vi "niWLAN - 80211abgnGeneration(ref).vi"(0 "Waveform Generation Settings":T1[](array[typedef])=[{"Standard"=0, "Channel Bandwidth (Hz)"=20000000.0, "Idle Interval (s)"=0.0001, "MCS Index"=0, "80211n PLCP Frame Format"=0, "Payload Data Length (bytes)"=100, "OFDM Data Rate (Mbps)"=0, "DSSS Data Rate (Mbps)"=0, "Wfm_Index"=0}, {"Standard"=0, "Channel Bandwidth (Hz)"=20000000.0, "Idle Interval (s)"=0.001, "MCS Index"=0, "80211n PLCP Frame Format"=0, "Payload Data Length (bytes)"=200, "OFDM Data Rate (Mbps)"=2, "DSSS Data Rate (Mbps)"=0, "Wfm_Index"=1}, {"Standard"=0, "Channel Bandwidth (Hz)"=20000000.0, "Idle Interval (s)"=0.0001, "MCS Index"=0, "80211n PLCP Frame Format"=0, "Payload Data Length (bytes)"=300, "OFDM Data Rate (Mbps)"=4, "DSSS Data Rate (Mbps)"=0, "Wfm_Index"=2}, {"Standard"=0, "Channel Bandwidth (Hz)"=20000000.0, "Idle Interval (s)"=0.0001, "MCS Index"=0, "80211n PLCP Frame Format"=0, "Payload Data Length (bytes)"=600, "OFDM Data Rate (Mbps)"=7, "DSSS Data Rate (Mbps)"=0, "Wfm_Index"=3}, {"Standard"=1, "Channel Bandwidth (Hz)"=20000000.0, "Idle Interval (s)"=0.0001, "MCS Index"=0, "80211n PLCP Frame Format"=0, "Payload Data Length (bytes)"=50, "OFDM Data Rate (Mbps)"=0, "DSSS Data Rate (Mbps)"=0, "Wfm_Index"=4}, {"Standard"=1, "Channel Bandwidth (Hz)"=20000000.0, "Idle Interval (s)"=0.0001, "MCS Index"=0, "80211n PLCP Frame Format"=0, "Payload Data Length (bytes)"=200, "OFDM Data Rate (Mbps)"=0, "DSSS Data Rate (Mbps)"=4, "Wfm_Index"=5}, {"Standard"=3, "Channel Bandwidth (Hz)"=20000000.0, "Idle Interval (s)"=0.0001, "MCS Index"=0, "80211n PLCP Frame Format"=0, "Payload Data Length (bytes)"=80, "OFDM Data Rate (Mbps)"=0, "DSSS Data Rate (Mbps)"=0, "Wfm_Index"=6}, {"Standard"=3, "Channel Bandwidth (Hz)"=20000000.0, "Idle Interval (s)"=0.0001, "MCS Index"=4, "80211n PLCP Frame Format"=0, "Payload Data Length (bytes)"=200, "OFDM Data Rate (Mbps)"=0, "DSSS Data Rate (Mbps)"=0, "Wfm_Index"=7}, {"Standard"=3, "Channel Bandwidth (Hz)"=20000000.0, "Idle Interval (s)"=0.0001, "MCS Index"=7, "80211n PLCP Frame Format"=0, "Payload Data Length (bytes)"=700, "OFDM Data Rate (Mbps)"=0, "DSSS Data Rate (Mbps)"=0, "Wfm_Index"=8}, {"Standard"=0, "Channel Bandwidth (Hz)"=20000000.0, "Idle Interval (s)"=0.0001, "MCS Index"=0, "80211n PLCP Frame Format"=0, "Payload Data Length (bytes)"=60, "OFDM Data Rate (Mbps)"=0, "DSSS Data Rate (Mbps)"=0, "Wfm_Index"=9}, {"Standard"=0, "Channel Bandwidth (Hz)"=20000000.0, "Idle Interval (s)"=0.0001, "MCS Index"=0, "80211n PLCP Frame Format"=0, "Payload Data Length (bytes)"=200, "OFDM Data Rate (Mbps)"=2, "DSSS Data Rate (Mbps)"=0, "Wfm_Index"=10}, {"Standard"=0, "Channel Bandwidth (Hz)"=20000000.0, "Idle Interval (s)"=0.0001, "MCS Index"=0, "80211n PLCP Frame Format"=0, "Payload Data Length (bytes)"=300, "OFDM Data Rate (Mbps)"=4, "DSSS Data Rate (Mbps)"=0, "Wfm_Index"=11}, {"Standard"=0, "Channel Bandwidth (Hz)"=20000000.0, "Idle Interval (s)"=0.0001, "MCS Index"=0, "80211n PLCP Frame Format"=0, "Payload Data Length (bytes)"=600, "OFDM Data Rate (Mbps)"=7, "DSSS Data Rate (Mbps)"=0, "Wfm_Index"=12}, {"Standard"=3, "Channel Bandwidth (Hz)"=20000000.0, "Idle Interval (s)"=0.0001, "MCS Index"=0, "80211n PLCP Frame Format"=0, "Payload Data Length (bytes)"=80, "OFDM Data Rate (Mbps)"=0, "DSSS Data Rate (Mbps)"=0, "Wfm_Index"=13}, {"Standard"=3, "Channel Bandwidth (Hz)"=20000000.0, "Idle Interval (s)"=0.0001, "MCS Index"=4, "80211n PLCP Frame Format"=0, "Payload Data Length (bytes)"=300, "OFDM Data Rate (Mbps)"=0, "DSSS Data Rate (Mbps)"=0, "Wfm_Index"=14}, {"Standard"=3, "Channel Bandwidth (Hz)"=20000000.0, "Idle Interval (s)"=0.0001, "MCS Index"=7, "80211n PLCP Frame Format"=0, "Payload Data Length (bytes)"=600, "OFDM Data Rate (Mbps)"=0, "DSSS Data Rate (Mbps)"=0, "Wfm_Index"=15}, {"Standard"=3, "Channel Bandwidth (Hz)"=40000000.0, "Idle Interval (s)"=0.0001, "MCS Index"=0, "80211n PLCP Frame Format"=0, "Payload Data Length (bytes)"=120, "OFDM Data Rate (Mbps)"=0, "DSSS Data Rate (Mbps)"=0, "Wfm_Index"=16}, {"Standard"=3, "Channel Bandwidth (Hz)"=40000000.0, "Idle Interval (s)"=0.0001, "MCS Index"=4, "80211n PLCP Frame Format"=0, "Payload Data Length (bytes)"=400, "OFDM Data Rate (Mbps)"=0, "DSSS Data Rate (Mbps)"=0, "Wfm_Index"=17}, {"Standard"=3, "Channel Bandwidth (Hz)"=40000000.0, "Idle Interval (s)"=0.0001, "MCS Index"=7, "80211n PLCP Frame Format"=0, "Payload Data Length (bytes)"=1024, "OFDM Data Rate (Mbps)"=0, "DSSS Data Rate (Mbps)"=0, "Wfm_Index"=18}] {"DSSS Data Rate (Mbps)" items=["1", "2", "5.5 CCK", "5.5 PBCC", "11 CCK", "11 PBCC", "22", "33"]; "OFDM Data Rate (Mbps)" items=["6", "9", "12", "18", "24", "36", "48", "54"]; "80211n PLCP Frame Format" items=["Mixed Format", "Greenfield Format"]; "Standard" items=["80211A/G/J/P OFDM", "80211B/G DSSS", "80211G DSSSOFDM", "80211N MIMOOFDM", "80211AC MIMOOFDM"]}, 5 "Without ACK ?":bool, 7 "Address String":string="00:90:4C:C5:12:38", 11 "error in":errorcluster) -> (4 "Output":T2(array[cluster]), 15 "error out":errorcluster)   [LabVIEW 2011]
uses:
  TV/RW/Includes/WLAN - TV - RW - INC - Rx_PER_Wfm_Settings.ctl
  <vilib>/RF Toolkits/WLAN/generation/controls/wlanG version control.ctl
  <vilib>/RF Toolkits/WLAN/generation/niWLANG Create Multiple Channel Waveform (IQ Complex Cluster).vi
  <vilib>/RF Toolkits/WLAN/generation/niWLANG Create Single Channel Waveform (IQ Complex Cluster).vi
  Program Files/National Instruments/LabVIEW 2011/resource/objmgr/niWLANGeneration.rc
panel:
  # "Hardware Configuration"
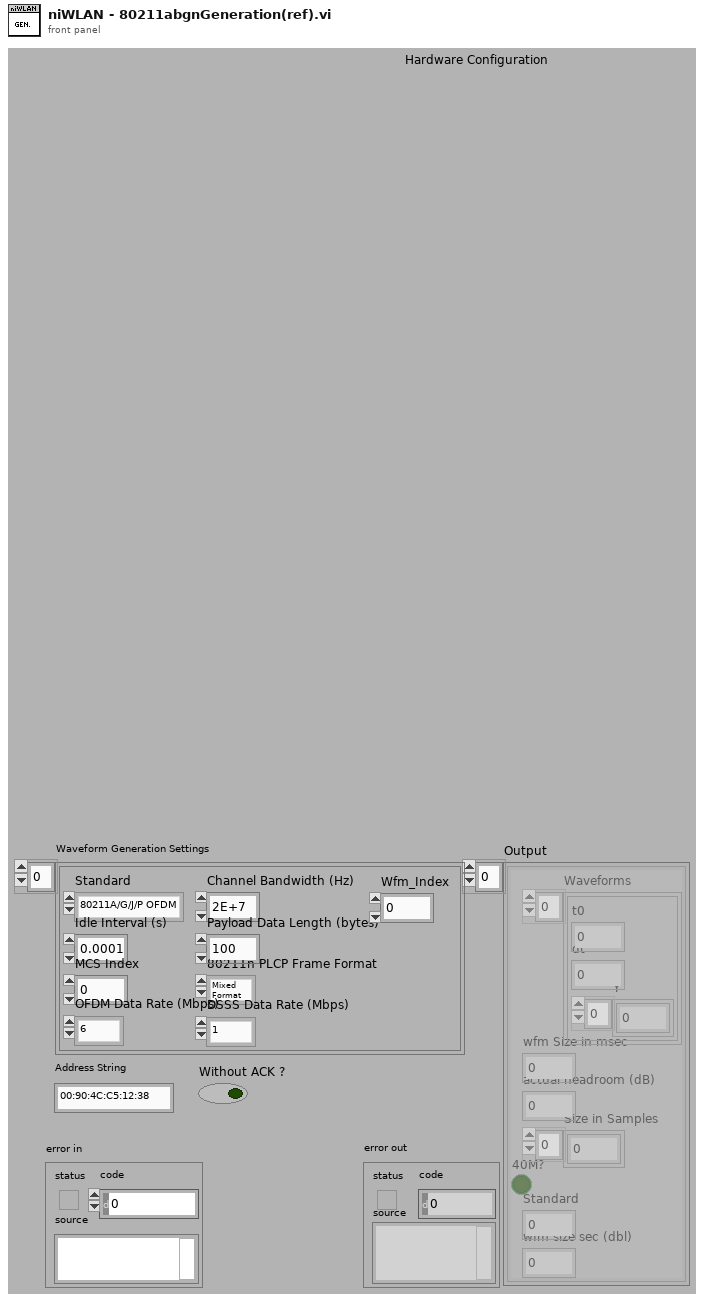
[diagram p1: front panel]
types:
  T1 = typedef "WLAN - TV - RW - INC - Rx_PER_Wfm_Settings.ctl" = cluster{"Standard":i32, "Channel Bandwidth (Hz)":dbl, "Idle Interval (s)":dbl, "MCS Index":i32, "80211n PLCP Frame Format":i32, "Payload Data Length (bytes)":i32, "OFDM Data Rate (Mbps)":i32, "DSSS Data Rate (Mbps)":i32, "Wfm_Index":i32}
  T2 = cluster{"Waveforms":cluster{"t0":dbl, "dt":dbl, "Y":cdb[]}[], "wfm Size in msec":i32, "actual headroom (dB)":dbl, "Size in Samples":i32[], "40M?":bool, "Standard ":i32, "wfm size sec (dbl)":dbl}[]
  T3 = cluster{"Waveforms":cluster{"t0":dbl, "dt":dbl, "Y":cdb[]}[], "wfm Size in msec":i32, "actual headroom (dB)":dbl, "Size in Samples":i32[], "40M?":bool, "Standard ":i32, "wfm size sec (dbl)":dbl}
  T4 = typedef "wlanG version control.ctl" = i32
  T5 = typedef "wlanv1_generation refnum.ctl" = refnum<k20>
  T6 = typedef "wlanv1_Generation Refnum.ctl" = refnum<k20>
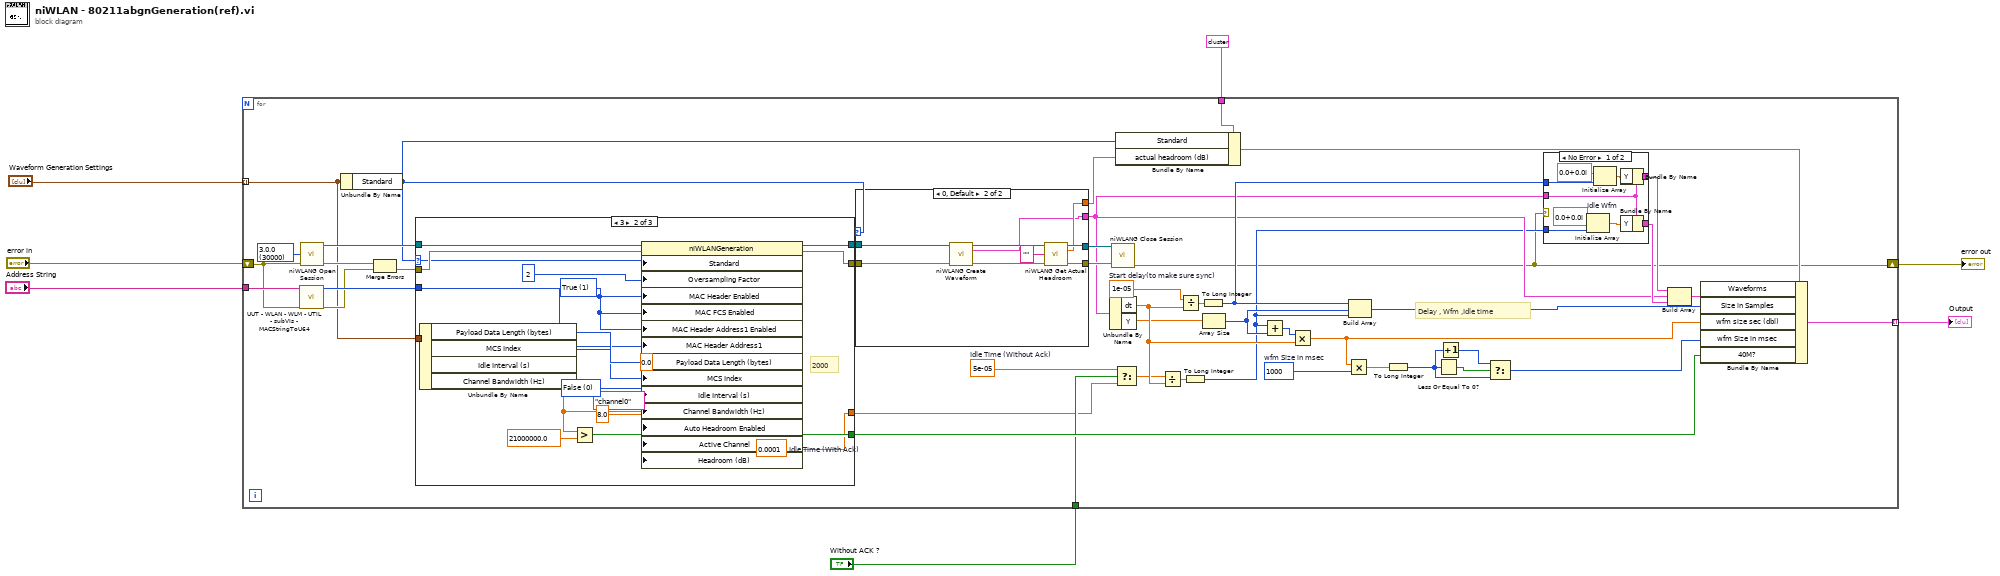
[diagram p0: block diagram]
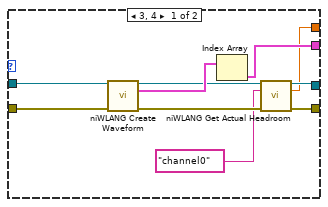
[diagram p3: hidden frame]
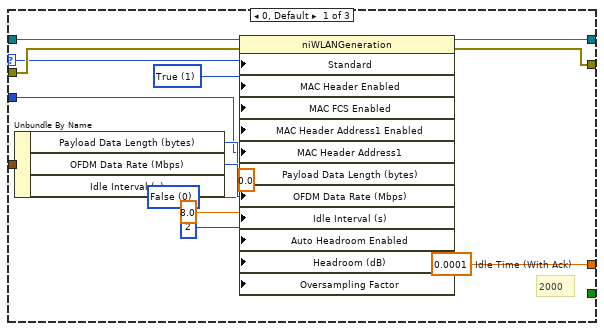
[diagram p4: hidden frame]
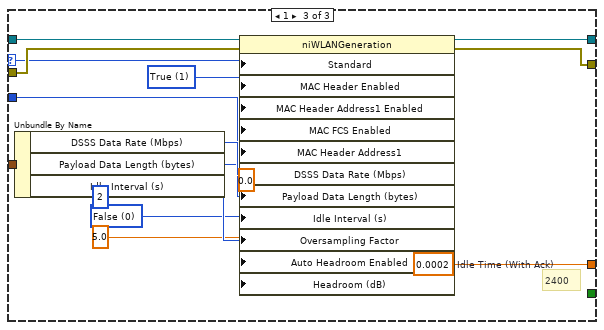
[diagram p5: hidden frame]
diagram:
  n1 = for {
    tunnel: "Address String" -> [w51]
    shift-right: [w8] -> w6
    shift-left: "error in" -> [w31]
    tunnel: T3 {"Waveforms"=[{"t0"=0.0, "dt"=1.25e-08, "Y"=array[800 elements]}, {"t0"=0.0, "dt"=1.25e-08, "Y"=array[85448 elements]}], "wfm Size in msec"=1, "actual headroom (dB)"=0.0, "Size in Samples"=[10000000, 0], "40M?"=TRUE, "Standard "=3, "wfm size sec (dbl)"=0.0} ("Cluster") -> [w15]
    tunnel: [w32] -> w3 mode=indexing
    tunnel: "Waveform Generation Settings" -> [w25] mode=indexing
    tunnel: "Without ACK ?" -> [w24]
    w21 = 1e-05  # Start delay(to make sure sync)
    w11 = 5e-05  # Idle Time (Without Ack)
    w49 = T4 30000 items=["1.0.0"=10000, "2.0.0"=20000, "3.0.0"=30000] ("toolkit compatibility version")
    w20 = 1000  # wfm Size in msec
    # "Delay , Wfm ,Idle time"
    n2 = call "UUT - WLAN - WLM - UTIL - subVIs - MACStringToU64.vi"("Address String"=w51, "error in"=w31) -> ("Address U64"=w52:u64, "error out"=w47:errorcluster)  [unwired: 12 in]
    n3 = call <vilib>:"niWLANG Open Session.vi"("toolkit compatibility version"=w49, "error in"=w31) -> ("niwlan generation session"=w50:T5, "error out"=w48:errorcluster)  [unwired: 11 in, 1 out]
    n4 = Unbundle By Name(w25) -> ("Standard"=w16:i32)
    n5 = Merge Errors(w48, w47) -> (w46:errorcluster)
    n6 = case shown="3" w16 {
      selector: w16 -> [w90 w109 w126]
      tunnel: w50 -> [w95 w113 w129]
      tunnel: w46 -> [w94 w110 w128]
      tunnel: [w93 w112 w127] -> w39
      tunnel: [w92 w111 w117] -> w38
      tunnel: w52 -> [w85 w102 w122]
      tunnel: w25 -> [w83 w106 w118]
      tunnel: [_ w98 _] -> w30
      tunnel: [w81 w96 w115] -> w9
      frame 0, Default {
        w81 = 0.0001  # Idle Time (With Ack)
        w88 = 0 items=["False", "True"] ("Auto Headroom Enabled")
        w91 = 1 items=["False", "True"] ("MAC Header Enabled")
        # "2000"
        n7 = Unbundle By Name(w83) -> ("Payload Data Length (bytes)"=w86:i32, "OFDM Data Rate (Mbps)"=w89:i32)  [unwired: 1 out]
        n8 = property class="niWLANGeneration"(reference=w95, error in=w94, "Standard"=w90, "MAC Header Enabled"=w91, "MAC FCS Enabled"=w91, "MAC Header Address1 Enabled"=w91, "MAC Header Address1"=w85, "Payload Data Length (bytes)"=w86, "OFDM Data Rate (Mbps)"=w89, "Idle Interval (s)"=0.0, "Auto Headroom Enabled"=w88, "Headroom (dB)"=8.0, "Oversampling Factor"=2) -> (reference out=w93:T5, error out=w92:errorcluster)
      }
      frame 3 {
        w96 = 0.0001  # Idle Time (With Ack)
        w105 = 0 items=["False", "True"] ("Auto Headroom Enabled")
        w114 = 1 items=["False", "True"] ("MAC Header Enabled")
        # "2000"
        n9 = Unbundle By Name(w106) -> ("Payload Data Length (bytes)"=w108:i32, "MCS Index"=w107:i32, "Channel Bandwidth (Hz)"=w101:dbl)  [unwired: 1 out]
        n10 = Greater?(x=w101, y=21000000.0) -> (0:w98:bool)
        n11 = property class="niWLANGeneration"(reference=w113, error in=w110, "Standard"=w109, "Oversampling Factor"=2, "MAC Header Enabled"=w114, "MAC FCS Enabled"=w114, "MAC Header Address1 Enabled"=w114, "MAC Header Address1"=w102, "Payload Data Length (bytes)"=w108, "MCS Index"=w107, "Idle Interval (s)"=0.0, "Channel Bandwidth (Hz)"=w101, "Auto Headroom Enabled"=w105, "Active Channel"="channel0", "Headroom (dB)"=8.0) -> (reference out=w112:T5, error out=w111:errorcluster)
      }
      frame 1 {
        w115 = 0.0002  # Idle Time (With Ack)
        w120 = 0 items=["False", "True"] ("Auto Headroom Enabled")
        w125 = 1 items=["False", "True"] ("OFDM Demod Enabled")
        # "2400"
        n12 = Unbundle By Name(w118) -> ("DSSS Data Rate (Mbps)"=w124:i32, "Payload Data Length (bytes)"=w123:i32)  [unwired: 1 out]
        n13 = property class="niWLANGeneration"(reference=w129, error in=w128, "Standard"=w126, "MAC Header Enabled"=w125, "MAC Header Address1 Enabled"=w125, "MAC FCS Enabled"=w125, "MAC Header Address1"=w122, "DSSS Data Rate (Mbps)"=w124, "Payload Data Length (bytes)"=w123, "Idle Interval (s)"=0.0, "Oversampling Factor"=2, "Auto Headroom Enabled"=w120, "Headroom (dB)"=5.0) -> (reference out=w127:T5, error out=w117:errorcluster)
      }
    }
    n14 = case shown="0, Default" w16 {
      tunnel: [w66 w80] -> w44
      tunnel: w39 -> [w70 w76]
      tunnel: w38 -> [w71 w75]
      tunnel: [w64 w79] -> w45
      tunnel: [w68 w72] -> w23
      tunnel: [w62 w78] -> w13
      frame 3, 4 {
        n15 = call-poly <vilib>:"niWLANG Create Waveform.vi"("niwlan generation session"=w70, "error in"=w71) -> ("niwlan generation session out"=w67:T6, "output waveform"=w69:cluster{"t0":dbl, "dt":dbl, "Y":cdb[]}[], "error out"=w65:errorcluster)  [unwired: 10 in, 1 out]
        n16 = Index Array(array=w69) -> (element=w68:cluster{"t0":dbl, "dt":dbl, "Y":cdb[]})  [unwired: 1 in]
        n17 = call <vilib>:"niWLANG Get Actual Headroom.vi"("niwlan generation session"=w67, "active channel"="channel0", "error in"=w65) -> ("niwlan generation session out"=w66:T6, "actual headroom (dB)"=w62:dbl, "error out"=w64:errorcluster)  [unwired: 10 in]
      }
      frame 0, Default {
        n18 = call-poly <vilib>:"niWLANG Create Waveform.vi"("niwlan generation session"=w76, "error in"=w75) -> ("niwlan generation session out"=w73:T5, "output waveform"=w72:cluster{"t0":dbl, "dt":dbl, "Y":cdb[]}, "error out"=w74:errorcluster)  [unwired: 10 in, 1 out]
        n19 = call <vilib>:"niWLANG Get Actual Headroom.vi"("niwlan generation session"=w73, "active channel"="", "error in"=w74) -> ("niwlan generation session out"=w80:T6, "actual headroom (dB)"=w78:dbl, "error out"=w79:errorcluster)  [unwired: 10 in]
      }
    }
    n20 = Unbundle By Name(w23) -> ("dt"=w22:dbl, "Y"=w17:cdb[])
    n21 = call <vilib>:"niWLANG Close Session.vi"("niwlan generation session"=w44, "error in"=w45) -> ("error out"=w8:errorcluster)  [unwired: 13 in]
    n22 = Bundle By Name(cluster=w15, "Standard"=w16, "actual headroom (dB)"=w13) -> (w14:T3)
    n23 = Select(t=w11, s=w24, f=w9) -> (s? t:f=w10:dbl)
    n24 = Divide(x=w10, y=w22) -> (x/y=w27:dbl)
    n25 = Divide(x=w21, y=w22) -> (x/y=w40:dbl)
    n26 = To Long Integer(number=w27) -> (32bit integer=w12:i32)
    n27 = To Long Integer(number=w40) -> (32bit integer=w37:i32)
    n28 = Array Size(array=w17) -> (size(s)=w28:i32)
    n29 = Add(x=w12, y=w28) -> (x+y=w26:i32)
    n30 = Multiply(x=w26, y=w22) -> (x*y=w18:dbl)
    n31 = Multiply(x=w18, y=w20) -> (x*y=w19:dbl)
    n32 = Build Array(w37, w28, w12) -> (w34:i32[])
    n33 = To Long Integer(number=w19) -> (32bit integer=w42:i32)
    n34 = Less Or Equal To 0?(x=w42) -> (x <= 0?=w43:bool)
    n35 = Increment(x=w42) -> (x+1=w41:i32)
    n36 = Select(t=w41, s=w43, f=w42) -> (s? t:f=w33:i32)
    n37 = case shown="No Error" w8 {
      tunnel: w37 -> [w61 _]
      tunnel: [w59 _] -> w36
      tunnel: [w56 _] -> w29
      tunnel: w23 -> [w55 _]
      tunnel: w12 -> [w53 _]
      frame No Error {
        n38 = Initialize Array "Idle Wfm"(cdb 0.0+0.0i ("element"), w53) -> (w57:cdb[])
        n39 = Initialize Array(cdb 0.0+0.0i ("element"), w61) -> (w60:cdb[])
        n40 = Bundle By Name(cluster=w55, "Y"=w60) -> (w59:cluster{"t0":dbl, "dt":dbl, "Y":cdb[]})
        n41 = Bundle By Name(cluster=w55, "Y"=w57) -> (w56:cluster{"t0":dbl, "dt":dbl, "Y":cdb[]})
      }
      frame Error {
      }
    }
    n42 = Build Array(w36, w23, w29) -> (w35:cluster{"t0":dbl, "dt":dbl, "Y":cdb[]}[])
    n43 = Bundle By Name(cluster=w14, "Waveforms"=w35, "Size in Samples"=w34, "wfm size sec (dbl)"=w18, "wfm Size in msec"=w33, "40M?"=w30) -> (w32:T3)
  }
  "error out" <- w6
  "Output" <- w3
